vi "监测块.vi"(10 "索引":i32, 11 "数组":u16[](array[numeric])) -> (1 "string":string, 2 "数值":sgl, 3 "time stamp":timestamp)   [LabVIEW 2016, in "CODCr库.lvlib"]
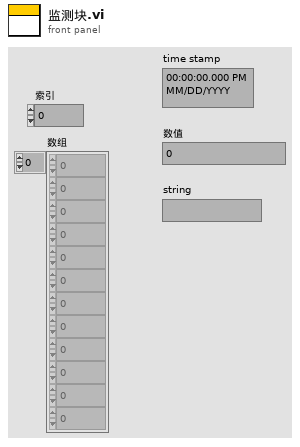
[diagram p1: front panel]
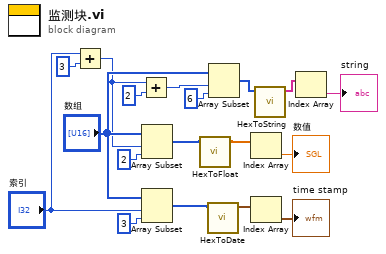
[diagram p0: block diagram]
diagram:
  n1 = Add(x="索引", y=3) -> (x+y=w9:i32)
  n2 = Add(x=w9, y=2) -> (x+y=w7:i32)
  n3 = Array Subset(array="数组", index=w9, length=2 ("长度")) -> (w6:u16[])
  n4 = Array Subset(array="数组", index="索引", length=3 ("长度")) -> (w2:u16[])
  n5 = call "HexToFloat.vi"("数组"=w6) -> ("FLOAT"=w5:sgl[])  [unwired: 10 in]
  n6 = call "HexToDate.vi"("数组"=w2) -> ("DATE"=w1:timestamp[])  [unwired: 10 in]
  n7 = Array Subset(array="数组", index=w7, length=6 ("长度")) -> (w4:u16[])
  n8 = Index Array(array=w5) -> (element=→"数值":sgl)  [unwired: 1 in]
  n9 = Index Array(array=w1) -> (element=→"time stamp":timestamp)  [unwired: 1 in]
  n10 = call "HexToString.vi"("数组"=w4) -> ("STRING"=w3:string[])  [unwired: 10 in]
  n11 = Index Array(array=w3) -> (element=→"string":string)  [unwired: 1 in]
